vi "UI Main.vi"() -> ()   [LabVIEW 2014]
uses:
  controls/Control Configuration.ctl
  controls/UI Data.ctl
  controls/All Control Configuration Values.ctl
  controls/Control State.ctl
  controls/Raw Values.ctl
  Globals/Global - All UI Loop Stop.vi
  Globals/Global - UI Stream and Variable Connections.vi
  Globals/Global - Configuration Options.vi
  support/User Event - Stop/User Event - Stop.lvlib
  support/Message Queue/Message Queue.lvlib
panel:
  in  "Switch to Safe State":bool
  in  "Exit":bool
  out "System Status":string
  out "Current Control Mode":u16(ring) items=["Safe State", "Manual", "Control (PID)"]
  in  "Settings Tab":T1(tab)
  in  "Channel 3 Setpoint":dbl
  in  "Channel 2 Setpoint":dbl
  in  "Channel 1 Setpoint":dbl
  in  "Channel 0 Setpoint":dbl
  in  "Update Control Configuration":bool
  in  "Control Configurations":T2[](array[typedef])
  in  "Run Control":bool
  in  "Stop Control":bool
  in  "Channel 3 Manual Value":dbl
  in  "Channel 2 Manual Value":dbl
  in  "Channel 1 Manual Value":dbl
  in  "Channel 0 Manual Value":dbl
  in  "Run Manual":bool
  in  "Stop Manual":bool
  out "Control Input Values":T3(graph)
  out "Control Output Values":T3(graph)
  out "Control Loop Period (ms)":u32
  out "Largest Contiguous Memory (bytes)":dbl(graph)
  out "CPU Usage (%)":dbl(graph)
  out "Connected?":bool
  in  "Connect to Controller":bool
  in  "Controller Address":string
  # "LabVIEW Real-Time Control (NI-DAQmx)"
  # "Connection Settings"
  # "Element 0 - Chan 0\nElement 1 - Chan 1\nElement 2 - Chan 2\nElement 3 - Chan 3"
  # "Setpoint changes are sent to the target automatically."
  # "Control Configuration changes are sent to the target when you click \"Update Control Configurations\"."
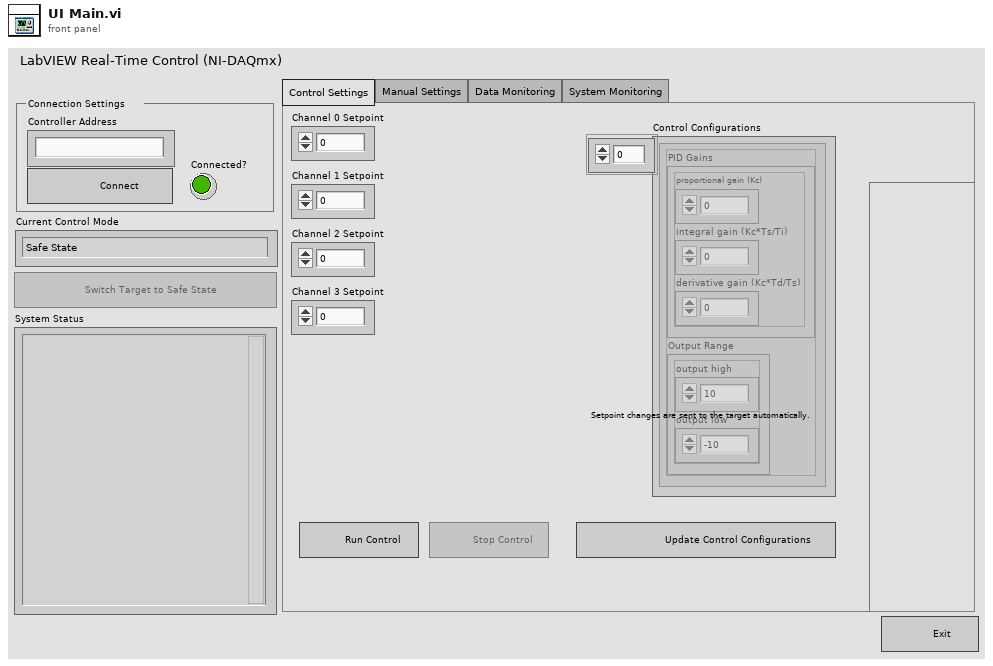
[diagram p1: front panel]
types:
  T1 = enum32{"Control Settings", "Manual Settings", "Data Monitoring", "System Monitoring"}
  T2 = typedef "Control Configuration.ctl" = cluster{"PID Gains":cluster{"proportional gain (Kc)":dbl, "integral gain (Kc*Ts/Ti)":dbl, "derivative gain (Kc*Td/Ts)":dbl}, "Output Range":cluster{"output high":dbl, "output low":dbl}}
  T3 = cluster{"Array of Double[0]":dbl, "Array of Double[1]":dbl, "Array of Double[2]":dbl, "Array of Double[3]":dbl}
  T4 = typedef "UI Data.ctl" = cluster{"Switch to Safe State Ref":refnum<vi>, "Run Manual Ref":refnum<vi>, "Stop Manual Ref":refnum<vi>, "Run Control Ref":refnum<vi>, "Stop Control Ref":refnum<vi>, "Update Control Configurations Ref":refnum<vi>, "Ch 0 Setpoint Ref":refnum<vi>, "Ch 1 Setpoint Ref":refnum<vi>, "Ch 2 Setpoint Ref":refnum<vi>, "Ch 3 Setpoint Ref":refnum<vi>, "Ch 0 Manual Ref":refnum<vi>, "Ch 1 Manual Ref":refnum<vi>, "Ch 2 Manual Ref":refnum<vi>, "Ch 3 Manual Ref":refnum<vi>, "Control Configurations Ref":refnum<vi>}
  T5 = typedef "Message Queue.lvlib/All Message Queues.ctl" = cluster{"UI":refnum<queue>}
  T6 = cluster{"Channel 0 Setpoint":dbl, "Channel 1 Setpoint":dbl, "Channel 2 Setpoint":dbl, "Channel 3 Setpoint":dbl}
  T7 = cluster{"Channel 0 Manual Value":dbl, "Channel 1 Manual Value":dbl, "Channel 2 Manual Value":dbl, "Channel 3 Manual Value":dbl}
  T8 = cluster{"Message":string, "Message Data":variant}
  T9 = typedef "All Control Configuration Values.ctl" = cluster{"Control State":T10, "Setpoints":T11, "Manual Values":T11, "Control Configurations":T2[]}
  T10 = typedef "Control State.ctl" = enum16{"Safe State", "Manual", "Control (PID)"}
  T11 = typedef "Raw Values.ctl" = cluster{"Channel 0":dbl, "Channel 1":dbl, "Channel 2":dbl, "Channel 3":dbl}
  T12 = typedef "Variable References.ctl" = cluster{"CPU Usage":refnum<k21>, "Contiguous Memory":refnum<k21>, "Control Mode":refnum<k21>, "Control Loop Period":refnum<k21>, "Input Values":refnum<k21>, "Output Values":refnum<k21>}
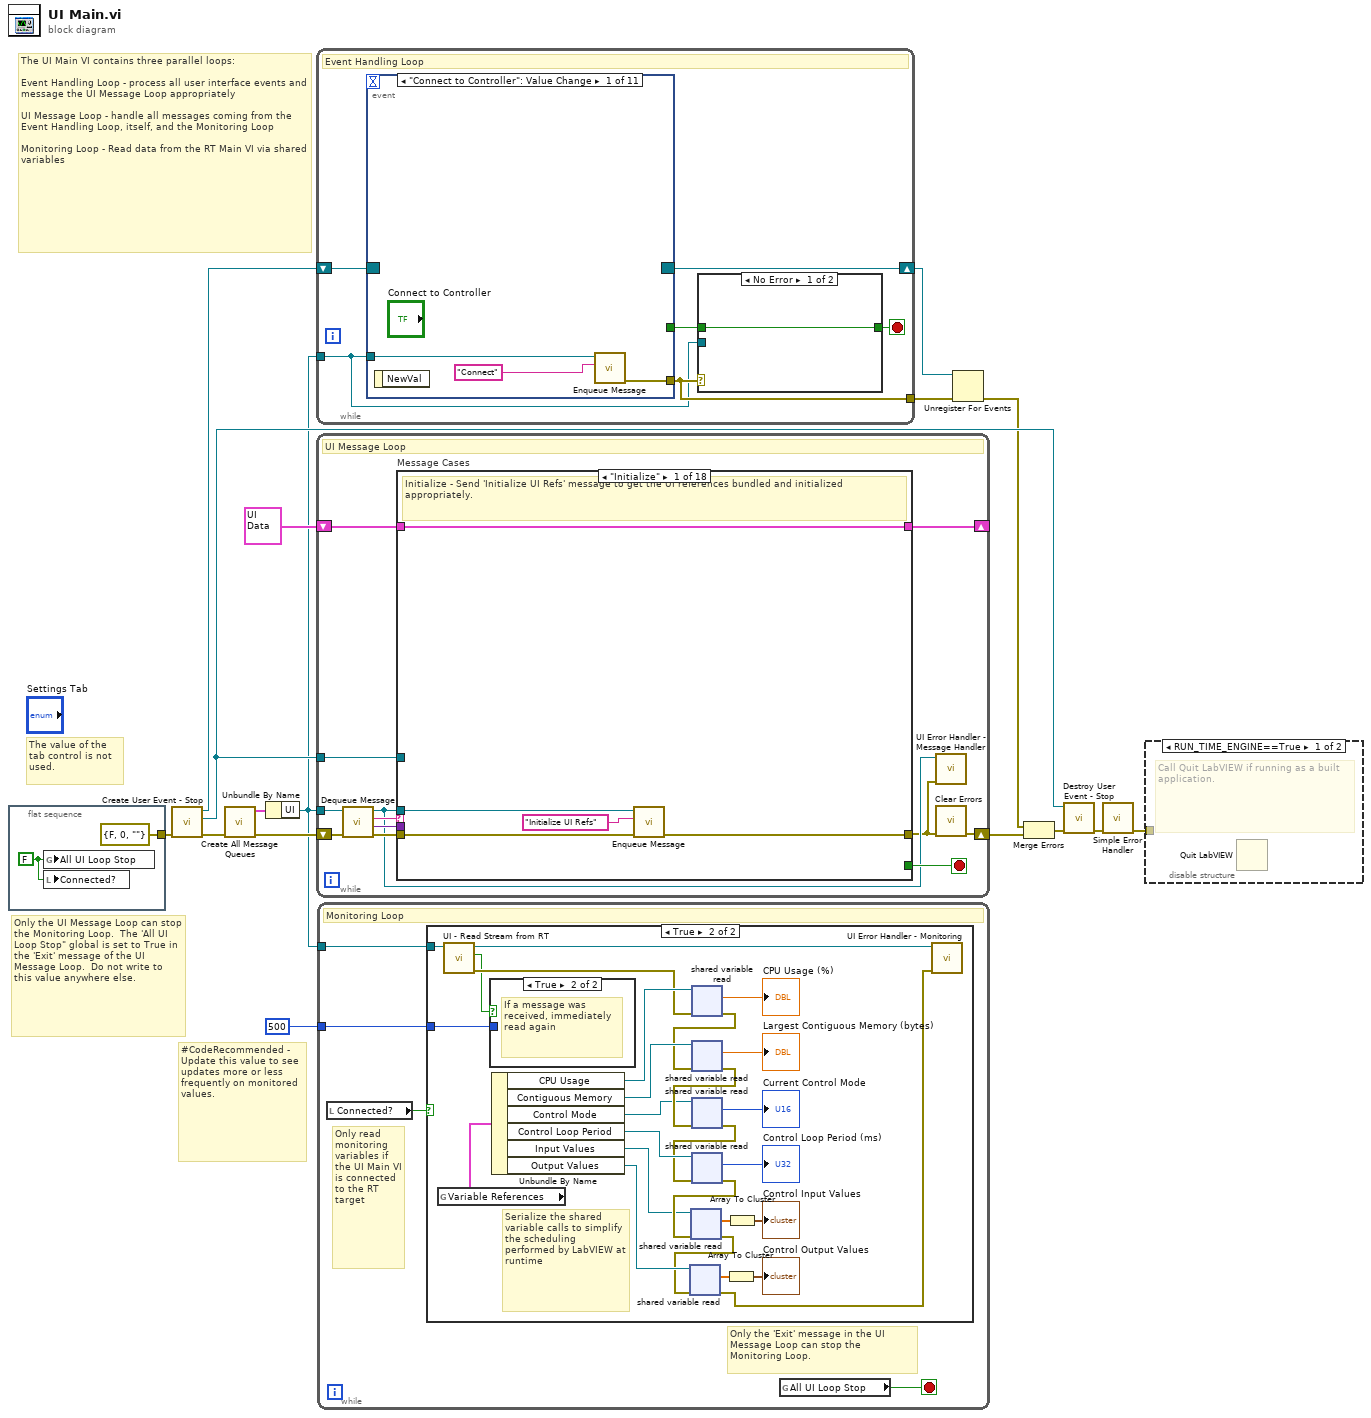
[diagram p0: block diagram]
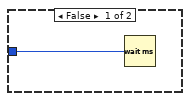
[diagram p3: hidden frame]
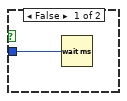
[diagram p4: hidden frame]
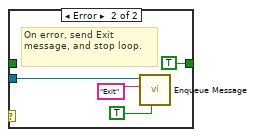
[diagram p5: hidden frame]
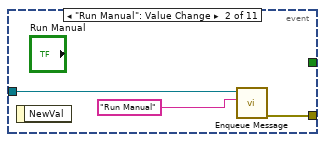
[diagram p6: hidden frame]
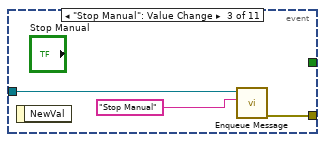
[diagram p7: hidden frame]
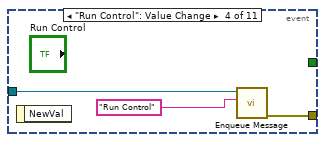
[diagram p8: hidden frame]
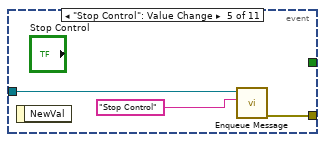
[diagram p9: hidden frame]
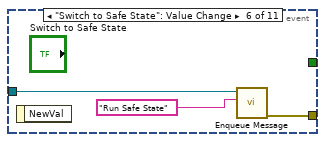
[diagram p10: hidden frame]
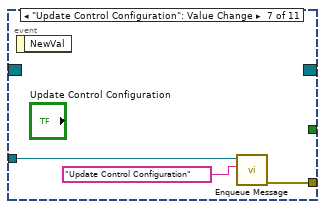
[diagram p11: hidden frame]
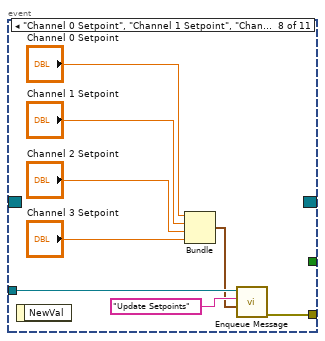
[diagram p12: hidden frame]
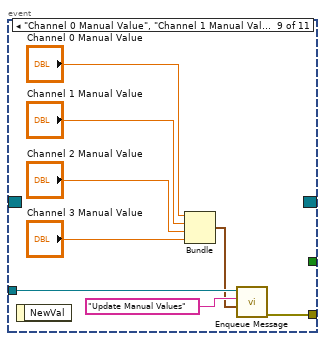
[diagram p13: hidden frame]
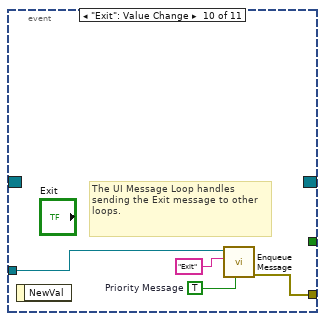
[diagram p14: hidden frame]
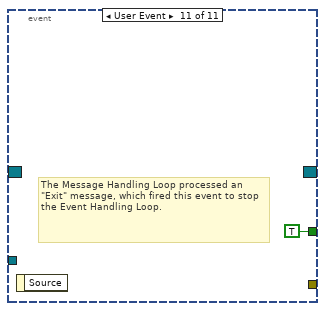
[diagram p15: hidden frame]
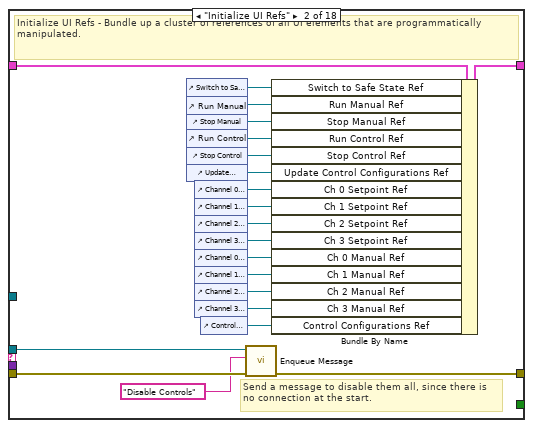
[diagram p16: hidden frame]
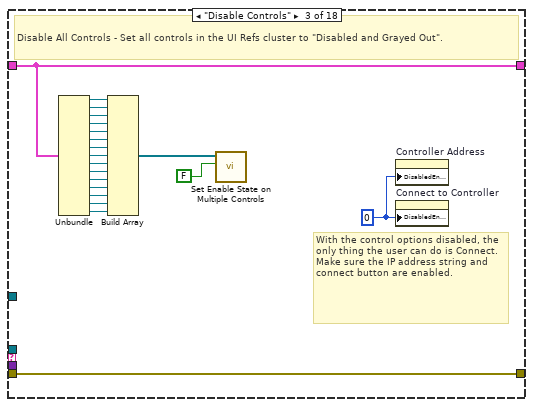
[diagram p17: hidden frame]
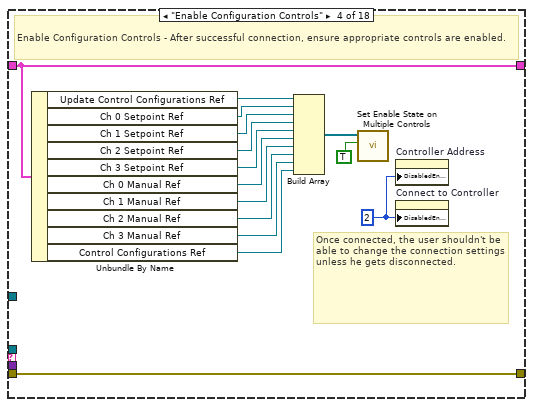
[diagram p18: hidden frame]
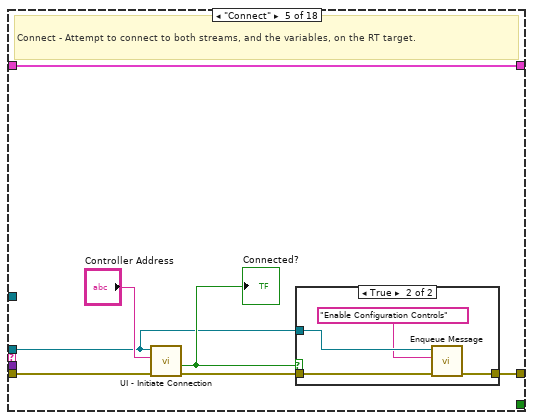
[diagram p19: hidden frame]
diagram:
  # "#CodeRecommended - Update this value to see updates more or less frequently on monitored values."
  # "The UI Main VI contains three parallel loops:\n\nEvent Handling Loop - process all user interface events and message the UI Message Loop appropriately\n\nUI Message Loop - handle all messages coming from the Event Handling Loop, itself, and the Monitoring Loop\n\nMonitoring Loop - Read data from the RT Main VI via shared variables"
  # "The value of the tab control is not used."
  # "Only the UI Message Loop can stop the Monitoring Loop.  The 'All UI Loop Stop\" global is set to True in the 'Exit' message of the UI Message Loop.  Do not write to this value anywhere else."
  n1 = flat-sequence {
    tunnel: [errorcluster {"status"=FALSE, "code"=0, "source"=""} ("error in (no error)")] -> w3
    frame #0 {
      w17 = FALSE
      n2 = global write "Global - All UI Loop Stop.vi" "All UI Loop Stop"(w17) -> ()
      n3 = local write "Connected?"(w17) -> ()
    }
  }
  n4 = call "Create User Event - Stop.vi"("error in (no error)"=w3) -> ("error out"=w11:errorcluster, "User Event - Stop"=w12:refnum<user-event>, "Stop Event Registration Refnum"=w13:refnum<event-registration>)  [unwired: 8 in]
  n5 = call "Create All Message Queues.vi"("error in (no error)"=w11) -> ("error out"=w9:errorcluster, "Message Queues out"=w10:T5)  [unwired: 9 in]
  n6 = Unbundle By Name(w10) -> ("UI"=w4:refnum<queue>)
  n7 = while {
    tunnel: w4 -> [w20]
    tunnel: [w22] -> w15
    shift-right: [w19] -> w7
    shift-left: w13 -> [w21]
    stop <- w23 stop-if-true
    # "Event Handling Loop"
    n8 = event shown="[0] \"Connect to Controller\": Value Change" {
      selector: w21 -> [_ _ _ _ _ _ _ _ _ _ _]
      dyn-events: [_ _ _ _ _ _ _ _ _ _ _] -> w19
      timeout: _ -> [_ _ _ _ _ _ _ _ _ _ _]
      tunnel: [_ _ _ _ _ _ _ _ _ _ TRUE ("Discard?")] -> w24
      tunnel: w20 -> [w30 w33 w36 w39 w42 w45 w50 w53 w65 w67 _]
      tunnel: [w32 w35 w38 w41 w44 w47 w49 w52 w64 w70 _] -> w22
      event "Connect to Controller": Value Change {
        n9 = event-data() -> ()  [unwired: 1 in, 1 out]
        n10 = call "Enqueue Message.vi"("Message"="Connect", "Message Queue"=w30) -> ("error out"=w32:errorcluster)  [unwired: 8 in, 1 out]
      }
      event "Run Manual": Value Change {
        n11 = event-data() -> ()  [unwired: 1 in, 1 out]
        n12 = call "Enqueue Message.vi"("Message"="Run Manual", "Message Queue"=w33) -> ("error out"=w35:errorcluster)  [unwired: 8 in, 1 out]
      }
      event "Stop Manual": Value Change {
        n13 = event-data() -> ()  [unwired: 1 in, 1 out]
        n14 = call "Enqueue Message.vi"("Message"="Stop Manual", "Message Queue"=w36) -> ("error out"=w38:errorcluster)  [unwired: 8 in, 1 out]
      }
      event "Run Control": Value Change {
        n15 = event-data() -> ()  [unwired: 1 in, 1 out]
        n16 = call "Enqueue Message.vi"("Message"="Run Control", "Message Queue"=w39) -> ("error out"=w41:errorcluster)  [unwired: 8 in, 1 out]
      }
      event "Stop Control": Value Change {
        n17 = event-data() -> ()  [unwired: 1 in, 1 out]
        n18 = call "Enqueue Message.vi"("Message"="Stop Control", "Message Queue"=w42) -> ("error out"=w44:errorcluster)  [unwired: 8 in, 1 out]
      }
      event "Switch to Safe State": Value Change {
        n19 = event-data() -> ()  [unwired: 1 in, 1 out]
        n20 = call "Enqueue Message.vi"("Message"="Run Safe State", "Message Queue"=w45) -> ("error out"=w47:errorcluster)  [unwired: 8 in, 1 out]
      }
      event "Update Control Configuration": Value Change {
        n21 = event-data() -> ()  [unwired: 1 in, 1 out]
        n22 = call "Enqueue Message.vi"("Message"="Update Control Configuration", "Message Queue"=w50) -> ("error out"=w49:errorcluster)  [unwired: 8 in, 1 out]
      }
      event "Channel 0 Setpoint", "Channel 1 Setpoint", "Channel 2 Setpoint", "Channel 3 Setpoint": Value Change {
        n23 = event-data() -> ()  [unwired: 1 in, 1 out]
        n24 = Bundle("Channel 0 Setpoint"="Channel 0 Setpoint", "Channel 1 Setpoint"="Channel 1 Setpoint", "Channel 2 Setpoint"="Channel 2 Setpoint", "Channel 3 Setpoint"="Channel 3 Setpoint") -> (w51:T6)  [unwired: 1 in]
        n25 = call "Enqueue Message.vi"("Message Data"=w51, "Message"="Update Setpoints", "Message Queue"=w53) -> ("error out"=w52:errorcluster)  [unwired: 7 in, 1 out]
      }
      event "Channel 0 Manual Value", "Channel 1 Manual Value", "Channel 2 Manual Value", "Channel 3 Manual Value": Value Change {
        n26 = event-data() -> ()  [unwired: 1 in, 1 out]
        n27 = Bundle("Channel 0 Manual Value"="Channel 0 Manual Value", "Channel 1 Manual Value"="Channel 1 Manual Value", "Channel 2 Manual Value"="Channel 2 Manual Value", "Channel 3 Manual Value"="Channel 3 Manual Value") -> (w63:T7)  [unwired: 1 in]
        n28 = call "Enqueue Message.vi"("Message Data"=w63, "Message"="Update Manual Values", "Message Queue"=w65) -> ("error out"=w64:errorcluster)  [unwired: 7 in, 1 out]
      }
      event "Exit": Value Change {
        w68 = TRUE  # Priority Message
        # "The UI Message Loop handles sending the Exit message to other loops."
        n29 = event-data() -> ()  [unwired: 1 in, 1 out]
        n30 = call "Enqueue Message.vi"("Priority Message? (F)"=w68, "Message"="Exit", "Message Queue"=w67) -> ("error out"=w70:errorcluster)  [unwired: 7 in, 1 out]
      }
      event User Event {
        # "The Message Handling Loop processed an \"Exit\" message, which fired this event to stop the Event Handling Loop."
        n31 = event-data() -> ()  [unwired: 1 in, 1 out]
      }
    }
    n32 = case shown="No Error" w22 {
      tunnel: [w25 TRUE ("Discard?")] -> w23
      tunnel: w24 -> [w25 _]
      tunnel: w20 -> [_ w26]
      frame No Error {
      }
      frame Error {
        # "On error, send Exit message, and stop loop."
        n33 = call "Enqueue Message.vi"("Priority Message? (F)"=TRUE ("Discard?"), "Message"="Exit", "Message Queue"=w26) -> ()  [unwired: 7 in, 2 out]
      }
    }
  }
  n34 = while {
    tunnel: w4 -> [w77]
    tunnel: w12 -> [w82]
    shift-right: [w72] -> w16
    shift-left: w9 -> [w81]
    shift-right: [w75] -> _
    shift-left: T4 {"Switch to Safe State Ref"=refnum, "Run Manual Ref"=refnum, "Stop Manual Ref"=refnum, "Run Control Ref"=refnum, "Stop Control Ref"=refnum, "Update Control Configurations Ref"=refnum, "Ch 0 Setpoint Ref"=refnum, "Ch 1 Setpoint Ref"=refnum, "Ch 2 Setpoint Ref"=refnum, "Ch 3 Setpoint Ref"=refnum, "Ch 0 Manual Ref"=refnum, "Ch 1 Manual Ref"=refnum, "Ch 2 Manual Ref"=refnum, "Ch 3 Manual Ref"=refnum, "Control Configurations Ref"=refnum} ("Measurement UI Controls") -> [w76]
    stop <- w83 stop-if-true
    # "UI Message Loop"
    n35 = call "Dequeue Message.vi"("error in (no error)"=w81, "Message Queue"=w77) -> ("error out"=w80:errorcluster, "Message Data"=w78:variant, "Message"=w79:string, "dup Message Queue"=w74:refnum<queue>)  [unwired: 6 in]
    n36 = case "Message Cases" shown="\"Initialize\"" w79 {
      selector: w79 -> [_ _ _ _ _ _ _ _ _ w206 _ w238 _ w288 _ _ _ w350]
      tunnel: w74 -> [w85 w97 _ _ w146 _ w164 _ w188 w207 _ _ _ w292 _ w335 _ _]
      tunnel: w80 -> [w87 w109 w129 w135 w151 w162 w166 w171 w202 w209 w227 w239 w252 w302 w323 w340 w345 _]
      tunnel: [w86 w98 w129 w135 w145 w162 w165 w170 w190 w208 w226 w240 w250 w303 w321 w341 w344 w348] -> w73
      tunnel: [_ _ _ _ _ _ _ _ _ _ _ _ _ _ _ TRUE _ _] -> w83
      tunnel: w78 -> [_ _ _ _ _ _ _ _ w200 _ _ w237 w251 w300 w320 _ _ _]
      tunnel: w82 -> [_ _ _ _ _ _ _ _ _ _ _ _ _ _ _ w339 _ _]
      tunnel: w76 -> [w88 w108 w128 w141 w150 w161 w168 w172 w197 w210 w228 w241 w249 w304 w322 w337 w343 w346]
      tunnel: [w88 w107 w128 w141 w150 w161 w168 w172 w197 w210 w228 w241 w249 w304 w322 w337 w343 w346] -> w75
      frame "Initialize" {
        # "Initialize - Send 'Initialize UI Refs' message to get the UI references bundled and initialized appropriately."
        n37 = call "Enqueue Message.vi"("error in (no error)"=w87, "Message"="Initialize UI Refs", "Message Queue"=w85) -> ("error out"=w86:errorcluster)  [unwired: 7 in, 1 out]
      }
      frame "Initialize UI Refs" {
        # "Send a message to disable them all, since there is no connection at the start."
        # "Initialize UI Refs - Bundle up a cluster of references of all UI elements that are programmatically manipulated."
        n38 = control-ref of="Switch to Safe State"() -> (w106:refnum<vi>)
        n39 = control-ref of="Run Manual"() -> (w90:refnum<vi>)
        n40 = control-ref of="Stop Manual"() -> (w89:refnum<vi>)
        n41 = control-ref of="Run Control"() -> (w105:refnum<vi>)
        n42 = control-ref of="Stop Control"() -> (w104:refnum<vi>)
        n43 = control-ref of="Update Control Configuration"() -> (w103:refnum<vi>)
        n44 = control-ref of="Channel 0 Setpoint"() -> (w102:refnum<vi>)
        n45 = control-ref of="Channel 1 Setpoint"() -> (w101:refnum<vi>)
        n46 = control-ref of="Channel 2 Setpoint"() -> (w100:refnum<vi>)
        n47 = control-ref of="Channel 3 Setpoint"() -> (w99:refnum<vi>)
        n48 = control-ref of="Channel 0 Manual Value"() -> (w94:refnum<vi>)
        n49 = control-ref of="Channel 1 Manual Value"() -> (w93:refnum<vi>)
        n50 = control-ref of="Channel 2 Manual Value"() -> (w92:refnum<vi>)
        n51 = control-ref of="Channel 3 Manual Value"() -> (w91:refnum<vi>)
        n52 = control-ref of="Control Configurations"() -> (w95:refnum<vi>)
        n53 = call "Enqueue Message.vi"("error in (no error)"=w109, "Message"="Disable Controls", "Message Queue"=w97) -> ("error out"=w98:errorcluster)  [unwired: 7 in, 1 out]
        n54 = Bundle By Name(cluster=w108, "Switch to Safe State Ref"=w106, "Run Manual Ref"=w90, "Stop Manual Ref"=w89, "Run Control Ref"=w105, "Stop Control Ref"=w104, "Update Control Configurations Ref"=w103, "Ch 0 Setpoint Ref"=w102, "Ch 1 Setpoint Ref"=w101, "Ch 2 Setpoint Ref"=w100, "Ch 3 Setpoint Ref"=w99, "Ch 0 Manual Ref"=w94, "Ch 1 Manual Ref"=w93, "Ch 2 Manual Ref"=w92, "Ch 3 Manual Ref"=w91, "Control Configurations Ref"=w95) -> (w107:T4)
      }
      frame "Disable Controls" {
        w116 = 0
        # "With the control options disabled, the only thing the user can do is Connect. Make sure the IP address string and connect button are enabled."
        # "Disable All Controls - Set all controls in the UI Refs cluster to \"Disabled and Grayed Out\"."
        n55 = Unbundle(w128) -> ("Switch to Safe State Ref"=w127:refnum<vi>, "Run Manual Ref"=w126:refnum<vi>, "Stop Manual Ref"=w125:refnum<vi>, "Run Control Ref"=w124:refnum<vi>, "Stop Control Ref"=w123:refnum<vi>, "Update Control Configurations Ref"=w122:refnum<vi>, "Ch 0 Setpoint Ref"=w121:refnum<vi>, "Ch 1 Setpoint Ref"=w120:refnum<vi>, "Ch 2 Setpoint Ref"=w119:refnum<vi>, "Ch 3 Setpoint Ref"=w115:refnum<vi>, "Ch 0 Manual Ref"=w114:refnum<vi>, "Ch 1 Manual Ref"=w113:refnum<vi>, "Ch 2 Manual Ref"=w112:refnum<vi>, "Ch 3 Manual Ref"=w111:refnum<vi>, "Control Configurations Ref"=w110:refnum<vi>)
        n56 = Build Array(w127, w126, w125, w124, w123, w122, w121, w120, w119, w115, w114, w113, w112, w111, w110) -> (w118:refnum<vi>[])
        n57 = call "Set Enable State on Multiple Controls.vi"("Enable?"=FALSE, "Controls"=w118) -> ()  [unwired: 10 in]
        n58 = property on="Controller Address" class="Str"("DisabledEnum"=w116) -> ()  [unwired: 2 in, 2 out]
        n59 = property on="Connect to Controller" class="Bool"("DisabledEnum"=w116) -> ()  [unwired: 2 in, 2 out]
      }
      frame "Enable Configuration Controls" {
        w142 = 2
        # "Once connected, the user shouldn't be able to change the connection settings unless he gets disconnected."
        # "Enable Configuration Controls - After successful connection, ensure appropriate controls are enabled."
        n60 = Unbundle By Name(w141) -> ("Update Control Configurations Ref"=w140:refnum<vi>, "Ch 0 Setpoint Ref"=w139:refnum<vi>, "Ch 1 Setpoint Ref"=w138:refnum<vi>, "Ch 2 Setpoint Ref"=w137:refnum<vi>, "Ch 3 Setpoint Ref"=w136:refnum<vi>, "Ch 0 Manual Ref"=w134:refnum<vi>, "Ch 1 Manual Ref"=w133:refnum<vi>, "Ch 2 Manual Ref"=w132:refnum<vi>, "Ch 3 Manual Ref"=w131:refnum<vi>, "Control Configurations Ref"=w130:refnum<vi>)
        n61 = Build Array(w140, w139, w138, w137, w136, w134, w133, w132, w131, w130) -> (w144:refnum<vi>[])
        n62 = call "Set Enable State on Multiple Controls.vi"("Enable?"=TRUE, "Controls"=w144) -> ()  [unwired: 10 in]
        n63 = property on="Controller Address" class="Str"("DisabledEnum"=w142) -> ()  [unwired: 2 in, 2 out]
        n64 = property on="Connect to Controller" class="Bool"("DisabledEnum"=w142) -> ()  [unwired: 2 in, 2 out]
      }
      frame "Connect" {
        # "Connect - Attempt to connect to both streams, and the variables, on the RT target."
        n65 = call "UI - Initiate Connection.vi"("error in (no error)"=w151, "Controller Address"="Controller Address", "Message Queue"=w146) -> ("error out"=w148:errorcluster, "Connected?"=w147:bool)  [unwired: 7 in]
        "Connected?" <- w147
        n66 = case shown="True" w147 {
          tunnel: w148 -> [w152 w156]
          tunnel: w146 -> [_ w155]
          tunnel: [w152 w154] -> w145
          frame False {
          }
          frame True {
            n67 = call "Enqueue Message.vi"("error in (no error)"=w156, "Message"="Enable Configuration Controls", "Message Queue"=w155) -> ("error out"=w154:errorcluster)  [unwired: 7 in, 1 out]
          }
        }
      }
      frame "Close Connections" {
        # "Close Connections - Close the connections shared with the Monitoring Loop."
        n68 = global read "Global - UI Stream and Variable Connections.vi" "UI Command Stream"() -> (w160:refnum<k21>)
        n69 = global read "Global - UI Stream and Variable Connections.vi" "RT Message Stream"() -> (w159:refnum<k21>)
        n70 = global read "Global - UI Stream and Variable Connections.vi" "Variable References"() -> (w158:T12)
        n71 = local write "Connected?"(FALSE ("Connected?")) -> ()
        n72 = Destroy Stream Endpoint(11:w160) -> ()  [unwired: 1 in, 1 out]
        n73 = Destroy Stream Endpoint(11:w159) -> ()  [unwired: 1 in, 1 out]
        n74 = call "Close Variable Connections.vi"("Variable References"=w158) -> ()  [unwired: 11 in]
      }
      frame "Disconnect UI" {
        # "Disconnect UI - Something has gone wrong with the connection. Reinitialize the UI to its disconnected state."
        n75 = local write "Connected?"(FALSE ("Connected?")) -> ()
        n76 = call "Enqueue Message.vi"("error in (no error)"=w166, "Message"="Disable Controls", "Message Queue"=w164) -> ("error out"=w165:errorcluster)  [unwired: 7 in, 1 out]
      }
      frame "Get Control Settings from RT" {
        # "Get Control Settings from RT - Send a command to the RT to retrieve all current control parameter values and send them back to the UI."
        n77 = local read "Connected?"() -> (w169:bool)
        n78 = case shown="True" w169 {
          tunnel: w171 -> [w173 w177]
          tunnel: [w173 w176] -> w170
          frame False {
            # "Don't bother trying to send a message to the RT system if UI Main VI isn't even connected"
          }
          frame True {
            n79 = global read "Global - UI Stream and Variable Connections.vi" "UI Command Stream"() -> (w174:refnum<k21>)
            n80 = shared-variable-write(w174, w177, T8 {"Message"="Send Control Configuration to UI", "Message Data"=variant} ("data in")) -> (w176:errorcluster)  [unwired: 1 in, 2 out]
          }
        }
      }
      frame "Initial UI Values" {
        # "Set values of all setpoint and manual controls via reference."
        # "Initial UI Values - These are the current control values from the RT Control Loop. They are used to initialize the panel of UI Main VI upon successful connection to the RT target."
        n81 = Variant To Data(error in=w202, type=T9 {"Control State"=enum."Safe State", "Setpoints"={"Channel 0"=0.0, "Channel 1"=0.0, "Channel 2"=0.0, "Channel 3"=0.0}, "Manual Values"={"Channel 0"=0.0, "Channel 1"=0.0, "Channel 2"=0.0, "Channel 3"=0.0}, "Control Configurations"=[]} ("All FPGA Configuration Values"), Variant=w200) -> (data=w198:T9, error out=w201:errorcluster)
        n82 = Unbundle By Name(w197) -> ("Ch 0 Setpoint Ref"=w196:refnum<vi>, "Ch 1 Setpoint Ref"=w195:refnum<vi>, "Ch 2 Setpoint Ref"=w194:refnum<vi>, "Ch 3 Setpoint Ref"=w193:refnum<vi>, "Ch 0 Manual Ref"=w186:refnum<vi>, "Ch 1 Manual Ref"=w185:refnum<vi>, "Ch 2 Manual Ref"=w184:refnum<vi>, "Ch 3 Manual Ref"=w183:refnum<vi>)
        n83 = Unbundle By Name(w198) -> ("Setpoints"=w182:T11, "Manual Values"=w181:T11, "Control Configurations"=w191:T2[], "Control State"=w187:T10)
        n84 = Build Array(w196, w195, w194, w193, w186, w185, w184, w183) -> (w192:refnum<vi>[])
        n85 = Cluster To Array(cluster=w182) -> (array=w180:dbl[])
        n86 = Cluster To Array(cluster=w181) -> (array=w179:dbl[])
        n87 = local write "Control Configurations"(w191) -> ()
        n88 = local write "Current Control Mode"(w187) -> ()
        n89 = Build Array (concatenate)(w180, w179) -> (w178:dbl[])
        n90 = for {
          tunnel: w192 -> [w204] mode=indexing
          tunnel: w178 -> [w203] mode=indexing
          n91 = property class="DigNum"(reference=w204, "Value"=w203) -> ()  [unwired: 1 in, 2 out]
        }
        n92 = call "Enqueue Message.vi"("error in (no error)"=w201, "Message Data"=w187, "Message"="Update Display Mode", "Message Queue"=w188) -> ("error out"=w190:errorcluster)  [unwired: 6 in, 1 out]
      }
      frame "Run Control", "Run Manual", "Run Safe State", "Stop Control", "Stop Manual" {
        # "Run/Stop buttons - Send a command to switch the RT control loop into the appropriate state. Send a message to update this UI to reflect the new state."
        n93 = local read "Connected?"() -> (w205:bool)
        n94 = case shown="True" w205 {
          tunnel: w209 -> [w211 w221]
          tunnel: [w211 w217] -> w208
          tunnel: w207 -> [_ w216]
          tunnel: w206 -> [_ w215]
          frame False {
            # "Don't bother trying to send a message to the RT system if UI Main VI isn't even connected"
          }
          frame True {
            # "Run Control switches into its respective states. Anything else switches to Safe State."
            n95 = case shown="\"Safe State\", \"Stop Control\", \"Stop Manual\", Default" w215 {
              tunnel: [Control_State."Safe State" ("FPGA State") Control_State."Control (PID)" ("FPGA State") Control_State."Manual" ("FPGA State")] -> w212
              frame "Safe State", "Stop Control", "Stop Manual", Default {
              }
              frame "Run Control" {
              }
              frame "Run Manual" {
              }
            }
            n96 = global read "Global - UI Stream and Variable Connections.vi" "UI Command Stream"() -> (w213:refnum<k21>)
            n97 = Bundle("Update Control State", "FPGA State"=w212) -> (w218:cluster{string, "FPGA State":T10})  [unwired: 1 in]
            n98 = shared-variable-write(w213, w221, w218) -> (w220:errorcluster)  [unwired: 1 in, 2 out]
            n99 = call "Enqueue Message.vi"("error in (no error)"=w220, "Message Data"=w212, "Message"="Update Display Mode", "Message Queue"=w216) -> ("error out"=w217:errorcluster)  [unwired: 6 in, 1 out]
          }
        }
      }
      frame "Update Control Configuration" {
        # "Update Control Configuration - Send all control configurations to RT."
        n100 = local read "Connected?"() -> (w225:bool)
        n101 = case shown="True" w225 {
          tunnel: w227 -> [w229 w235]
          tunnel: [w229 w234] -> w226
          frame False {
            # "Don't bother trying to send a message to the RT system if UI Main VI isn't even connected"
          }
          frame True {
            n102 = global read "Global - UI Stream and Variable Connections.vi" "UI Command Stream"() -> (w230:refnum<k21>)
            n103 = Bundle("Update Control Configurations", "Control Configurations"="Control Configurations") -> (w232:cluster{string, "Control Configurations":T2[]})  [unwired: 1 in]
            n104 = shared-variable-write(w230, w235, w232) -> (w234:errorcluster)  [unwired: 1 in, 2 out]
          }
        }
      }
      frame "Update Manual Values", "Update Setpoints" {
        # "Update Setpoints/Manual Values - Send all setpoints/manual values to RT."
        n105 = local read "Connected?"() -> (w236:bool)
        n106 = case shown="True" w236 {
          tunnel: [w242 w248] -> w240
          tunnel: w239 -> [w242 w246]
          tunnel: w238 -> [_ w245]
          tunnel: w237 -> [_ w244]
          frame False {
            # "Don't bother trying to send a message to the RT system if UI Main VI isn't even connected"
          }
          frame True {
            n107 = global read "Global - UI Stream and Variable Connections.vi" "UI Command Stream"() -> (w243:refnum<k21>)
            n108 = Bundle(w245, "Message Data"=w244) -> (w247:cluster{string, "Message Data":variant})  [unwired: 1 in]
            n109 = shared-variable-write(w243, w246, w247) -> (w248:errorcluster)  [unwired: 1 in, 2 out]
          }
        }
      }
      frame "Update Display Mode" {
        # "Update Display Mode - Enable/Disable Controls appropriately for the new display mode."
        n110 = Variant To Data(error in=w252, type=Control_State."Safe State" ("Control State"), Variant=w251) -> (data=w259:T10, error out=w250:errorcluster)
        n111 = Unbundle By Name(w249) -> ("Switch to Safe State Ref"=w258:refnum<vi>, "Run Manual Ref"=w257:refnum<vi>, "Stop Manual Ref"=w256:refnum<vi>, "Run Control Ref"=w255:refnum<vi>, "Stop Control Ref"=w254:refnum<vi>)
        n112 = case shown="\"Control (PID)\"" w259 {
          tunnel: w258 -> [w264 w273 w280]
          tunnel: w257 -> [w260 w272 w282]
          tunnel: w256 -> [w263 w271 w279]
          tunnel: w255 -> [w262 w269 w281]
          tunnel: w254 -> [w261 w270 w278]
          frame "Control (PID)" {
            n113 = Build Array "Controls to Enable"(w264, w261, w260) -> (w268:refnum<vi>[])
            n114 = Build Array "Controls to Disable"(w263, w262) -> (w266:refnum<vi>[])
            n115 = call "Set Enable State on Multiple Controls.vi"("Enable?"=FALSE, "Controls"=w266) -> ()  [unwired: 10 in]
            n116 = call "Set Enable State on Multiple Controls.vi"("Enable?"=TRUE, "Controls"=w268) -> ()  [unwired: 10 in]
          }
          frame "Manual" {
            n117 = Build Array "Controls to Enable"(w273, w271, w269) -> (w277:refnum<vi>[])
            n118 = Build Array "Controls to Disable"(w272, w270) -> (w275:refnum<vi>[])
            n119 = call "Set Enable State on Multiple Controls.vi"("Enable?"=FALSE, "Controls"=w275) -> ()  [unwired: 10 in]
            n120 = call "Set Enable State on Multiple Controls.vi"("Enable?"=TRUE, "Controls"=w277) -> ()  [unwired: 10 in]
          }
          frame "Safe State" {
            # "This frame runs when the Control loop is in Safe State. Only enable the two run buttons."
            n121 = Build Array "Controls to Enable"(w282, w281) -> (w286:refnum<vi>[])
            n122 = Build Array "Controls to Disable"(w280, w279, w278) -> (w284:refnum<vi>[])
            n123 = call "Set Enable State on Multiple Controls.vi"("Enable?"=FALSE, "Controls"=w284) -> ()  [unwired: 10 in]
            n124 = call "Set Enable State on Multiple Controls.vi"("Enable?"=TRUE, "Controls"=w286) -> ()  [unwired: 10 in]
          }
        }
      }
      frame "Critical Error", "Log-Only Error", "Non-Critical Error", "RT Error" {
        # "Error - Display message in status indicator on panel.  If it's a critical error, shut down this VI with an 'Exit' message."
        n125 = case shown="Default" w288 {
          selector: w288 -> [_ w306]
          tunnel: ["UI Error" w306] -> w287
          frame Default {
          }
          frame "RT Error" {
          }
        }
        n126 = Variant To Data(error in=w302, type=errorcluster {"status"=FALSE, "code"=0, "source"=""} ("error constant"), Variant=w300) -> (data=w295:errorcluster, error out=w301:errorcluster)
        n127 = Unbundle By Name(w295) -> ("code"=w294:i32, "source"=w298:string)
        n128 = Format Date/Time String() -> (date/time string=w297:string)  [unwired: 3 in]
        n129 = Format Into String(format string="\n%s: %s %d - %s", w297, w287, w294, w298) -> (resulting string=w289:string)  [unwired: 2 in, 1 out]
        n130 = call "Enqueue Message.vi"("error in (no error)"=w301, "Message Data"=w289, "Message"="Update System Status", "Message Queue"=w292) -> ("error out"=w293:errorcluster, "dup Message Queue"=w291:refnum<queue>)  [unwired: 6 in]
        n131 = case shown="Default" w288 {
          tunnel: w293 -> [w307 w311]
          tunnel: w291 -> [_ w309]
          tunnel: [w307 w310] -> w303
          frame Default {
          }
          frame "Critical Error" {
            n132 = call "Enqueue Message.vi"("error in (no error)"=w311, "Message"="Exit", "Message Queue"=w309) -> ("error out"=w310:errorcluster)  [unwired: 7 in, 1 out]
          }
        }
      }
      frame "Update System Status" {
        # "#CodeRecommended - The code below ensures that the System Status string value does not become too large.  It uses the same maximum size as the RT error log to determine whether or not to remove the last half of the log string. Change this logic if you wish to maintain more/less of the information in the System Status string."
        # "Update System Status - Add a new string to the beginning of the System Status string on the UI."
        n133 = Variant To Data(error in=w323, type="", Variant=w320) -> (data=w317:string, error out=w321:errorcluster)
        n134 = local read "System Status"() -> (w315:string)
        n135 = global read "Global - Configuration Options.vi" "Error Log Max Size (bytes)"() -> (w313:i64)
        n136 = String Length(string=w315) -> (length=w316:i32)
        n137 = Greater?(x=w316, y=w313) -> (0:w314:bool)
        n138 = case shown="True" w314 {
          tunnel: w315 -> [w324 w328]
          tunnel: w313 -> [_ w327]
          tunnel: [w324 w329] -> w312
          frame False {
          }
          frame True {
            n139 = Divide(x=w327, y=i64 2) -> (x/y=w326:dbl)
            n140 = String Subset(string=w328, length (rest)=w326) -> (substring=w329:string)  [unwired: 1 in]
          }
        }
        n141 = Concatenate Strings(w317, w312) -> (→"System Status":string)
      }
      frame "Exit" {
        # "Flush the Writer Stream to ensure all pending messages are sent to RT Main VI"
        # "Close all connections"
        # "Stop Monitoring Loop"
        # "Stop Event Handling Loop"
        # "Release the UI Message queue reference"
        # "Stop UI Message Loop"
        # "Exit - Fire the User Event to stop the Event Handling Loop, and toggle the global variable to stop the Monitoring Loop.  This message alone causes all three loops to stop."
        n142 = global write "Global - All UI Loop Stop.vi" "All UI Loop Stop"(TRUE ("Stop Monitoring Loop")) -> ()
        n143 = call "Fire User Event - Stop.vi"("User Event - Stop"=w339) -> ("error out"=w338:errorcluster)  [unwired: 10 in]
        n144 = Release Queue(queue=w335, error in (no error)=w340) -> (error out=w336:errorcluster)  [unwired: 1 in, 2 out]
        n145 = global read "Global - UI Stream and Variable Connections.vi" "UI Command Stream"() -> (w331:refnum<k21>)
        n146 = global read "Global - UI Stream and Variable Connections.vi" "RT Message Stream"() -> (w333:refnum<k21>)
        n147 = global read "Global - UI Stream and Variable Connections.vi" "Variable References"() -> (w332:T12)
        n148 = Flush Stream(11:w331) -> (3:w330:refnum<k21>)  [unwired: 3 in, 2 out]
        n149 = Destroy Stream Endpoint(11:w333) -> ()  [unwired: 1 in, 1 out]
        n150 = call "Close Variable Connections.vi"("Variable References"=w332) -> ()  [unwired: 11 in]
        n151 = Destroy Stream Endpoint(11:w330) -> ()  [unwired: 1 in, 1 out]
        n152 = Merge Errors(w338, w336) -> (w341:errorcluster)
      }
      frame "---Copy This Frame---" {
        # "Duplicate this frame when creating new messages.  Change this comment in the duplicated frame to describe this message."
        n153 = Merge Errors(w345) -> (w344:errorcluster)
      }
      frame Default {
        # "'Default' case only runs if there is a message that isn't defined in any of the other cases.  Output a programming error."
        n154 = Format Into String(format string="The invalid message string \"%s\" was received in the Message Handling Loop." ("Invalid Message Loop Message"), w350) -> (resulting string=w347:string)  [unwired: 2 in, 1 out]
        n155 = call <vilib>:"Error Cluster From Error Code.vi"("error message (\"\")"=w347, "error code (0)"=1) -> ("error out"=w348:errorcluster)  [unwired: 7 in]
      }
    }
    n156 = call "UI Error Handler - Message Handler.vi"("error in (no error)"=w73, "Message Queue"=w74) -> ()  [unwired: 9 in, 1 out]
    n157 = call <vilib>:"Clear Errors.vi"("error in (no error)"=w73) -> ("error out"=w72:errorcluster)  [unwired: 5 in, 1 out]
  }
  n158 = while {
    tunnel: w4 -> [w354]
    tunnel: u32 500 ("milliseconds to wait") -> [w352]
    stop <- w355 stop-if-true
    # "Only read monitoring variables if the UI Main VI is connected to the RT target"
    # "Only the 'Exit' message in the UI Message Loop can stop the Monitoring Loop."
    # "Monitoring Loop"
    n159 = local read "Connected?"() -> (w353:bool)
    n160 = case shown="True" w353 {
      tunnel: w354 -> [_ w373]
      tunnel: w352 -> [w356 w368]
      frame False {
        n161 = Wait (ms)(milliseconds to wait=w356) -> ()  [unwired: 1 out]
      }
      frame True {
        # "Serialize the shared variable calls to simplify the scheduling performed by LabVIEW at runtime"
        n162 = global read "Global - UI Stream and Variable Connections.vi" "Variable References"() -> (w371:T12)
        n163 = call "UI - Read Stream from RT.vi"("Message Queue"=w373) -> ("error out"=w376:errorcluster, "Message Received?"=w369:bool, "dup Message Queue"=w372:refnum<queue>)  [unwired: 8 in]
        n164 = case shown="True" w369 {
          tunnel: w368 -> [w383 _]
          frame False {
            n165 = Wait (ms)(milliseconds to wait=w383) -> ()  [unwired: 1 out]
          }
          frame True {
            # "If a message was received, immediately read again"
          }
        }
        n166 = Unbundle By Name(w371) -> ("CPU Usage"=w379:refnum<k21>, "Contiguous Memory"=w378:refnum<k21>, "Control Mode"=w366:refnum<k21>, "Control Loop Period"=w377:refnum<k21>, "Input Values"=w364:refnum<k21>, "Output Values"=w362:refnum<k21>)
        n167 = shared-variable-read(w379, w376) -> (w375:errorcluster, →"CPU Usage (%)":dbl)  [unwired: 2 out]
        n168 = shared-variable-read(w378, w375) -> (w367:errorcluster, →"Largest Contiguous Memory (bytes)":dbl)  [unwired: 2 out]
        n169 = shared-variable-read(w366, w367) -> (w374:errorcluster, →"Current Control Mode":T10)  [unwired: 2 out]
        n170 = shared-variable-read(w377, w374) -> (w365:errorcluster, →"Control Loop Period (ms)":u32)  [unwired: 2 out]
        n171 = shared-variable-read(w364, w365) -> (w361:errorcluster, w363:dbl[])  [unwired: 2 out]
        n172 = shared-variable-read(w362, w361) -> (w359:errorcluster, w360:dbl[])  [unwired: 2 out]
        n173 = Array To Cluster(array=w360) -> (cluster=→"Control Output Values":T3)
        n174 = Array To Cluster(array=w363) -> (cluster=→"Control Input Values":T3)
        n175 = call "UI Error Handler - Monitoring.vi"("error in (no error)"=w359, "Message Queue"=w372) -> ()  [unwired: 9 in, 1 out]
      }
    }
    n176 = global read "Global - All UI Loop Stop.vi" "All UI Loop Stop"() -> (w355:bool)
  }
  n177 = Unregister For Events(event registration refnum=w7, error in=w15) -> (error out=w8:errorcluster)
  n178 = Merge Errors(w8, w16) -> (w14:errorcluster)
  n179 = call "Destroy User Event - Stop.vi"("error in (no error)"=w14, "User Event - Stop"=w12) -> ("error out"=w5:errorcluster)  [unwired: 9 in]
  n180 = call <vilib>:"Simple Error Handler.vi"("error in (no error)"=w5) -> ("error out"=w1:errorcluster)  [unwired: 4 in, 4 out]
  n181 = disable-structure shown="RUN_TIME_ENGINE==True" {
    disable-tunnel: w1 -> [_ _]
    frame condition #0 {
      # "Call Quit LabVIEW if running as a built application."
      n182 = Quit LabVIEW() -> ()  [unwired: 1 in]
    }
    frame condition #1 (active) {
    }
  }
